vi "Generate CD Storage Library Loader Path.vi"() -> (0 "CDS Loader path":path)   [LabVIEW 2019, in "DMA Channel Testing.lvclass"]
uses:
  DMA Channel Testing.lvclass
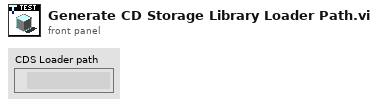
[diagram p1: front panel]
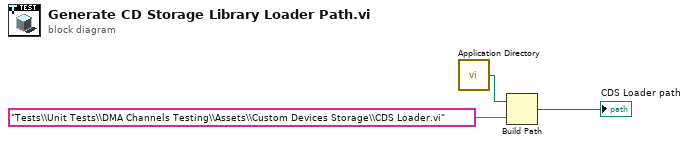
[diagram p0: block diagram]
diagram:
  n1 = call <vilib>:"Application Directory.vi"() -> ("Application Directory"=w1:path)
  n2 = Build Path(base path=w1, name or relative path="Tests\\Unit Tests\\DMA Channels Testing\\Assets\\Custom Devices Storage\\CDS Loader.vi") -> (appended path=→"CDS Loader path":path)
